vi "Show Block Diagram Event.vi"(8 "error in":errorcluster) -> (0 "error out":errorcluster)   [LabVIEW 2014, in "Chart Module.lvlib"]
uses:
  Chart Module.lvlib
  Show Block Diagram Argument--cluster.ctl
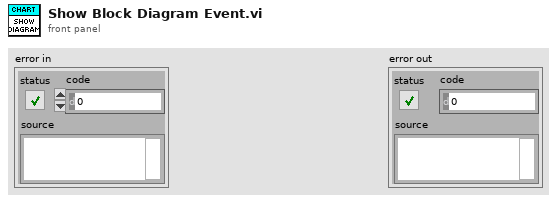
[diagram p1: front panel]
types:
  T1 = typedef "Chart Module.lvlib/Show Block Diagram Argument--cluster.ctl" = cluster{"Show Block Diagram?":bool}
  T2 = typedef "Chart Module.lvlib/Request Events--cluster.ctl" = cluster{"Stop Module":refnum<user-event>, "Show Panel":refnum<user-event>, "Hide Panel":refnum<user-event>, "Update Limits":refnum<user-event>, "Send Value":refnum<user-event>, "Clear Chart":refnum<user-event>, "Show Block Diagram":refnum<user-event>}
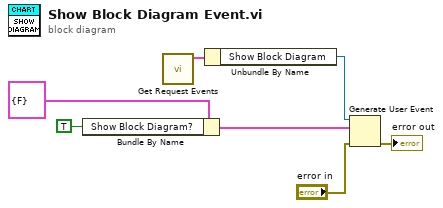
[diagram p0: block diagram]
diagram:
  n1 = Bundle By Name(cluster=T1 {"Show Block Diagram?"=FALSE} ("event data"), "Show Block Diagram?"=TRUE) -> (w4:T1)
  n2 = call "Get Request Events.vi"() -> ("Request Events"=w7:T2)  [unwired: 10 in, 1 out]
  n3 = Unbundle By Name(w7) -> ("Show Block Diagram"=w6:refnum<user-event>)
  n4 = Generate User Event(user event=w6, event data cluster=w4, error in="error in") -> (error out=→"error out":errorcluster)  [unwired: 1 in, 1 out]
